vi "Half Speed Converter.vi"(2 "Enable":bool, 3 "Y axis":dbl, 4 "X axis":dbl) -> (0 "Y axis":dbl, 1 "X axis":dbl)   [LabVIEW 2014]
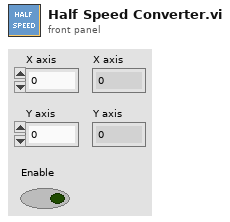
[diagram p1: front panel]
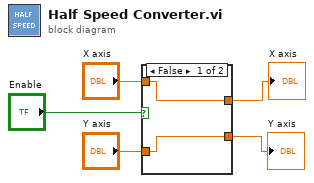
[diagram p0: block diagram]
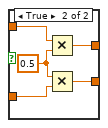
[diagram p2: hidden frame]
diagram:
  n1 = case shown="False" "Enable" {
    tunnel: "X axis" -> [w7 w11]
    tunnel: "Y axis" -> [w6 w10]
    tunnel: [w6 w9] -> w3
    tunnel: [w7 w8] -> w2
    frame False {
    }
    frame True {
      w12 = 0.5 ("x")
      n2 = Multiply(x=w11, y=w12) -> (x*y=w8:dbl)
      n3 = Multiply(x=w12, y=w10) -> (x*y=w9:dbl)
    }
  }
  "X axis" <- w2
  "Y axis" <- w3
